vi "Read VI Ref.vi"(8 "error in (no error)":errorcluster, 11 "Graph in":refnum<class "Graph.lvclass">) -> (0 "error out":errorcluster, 2 "VI Ref":refnum<vi>, 3 "Graph out":refnum<class "Graph.lvclass">)   [LabVIEW 2021, in "Graph.lvclass"]
doc: "This vi reads Graph VI Refs."
uses:
  Graph.lvclass
  Graph.lvclass/Graph.ctl
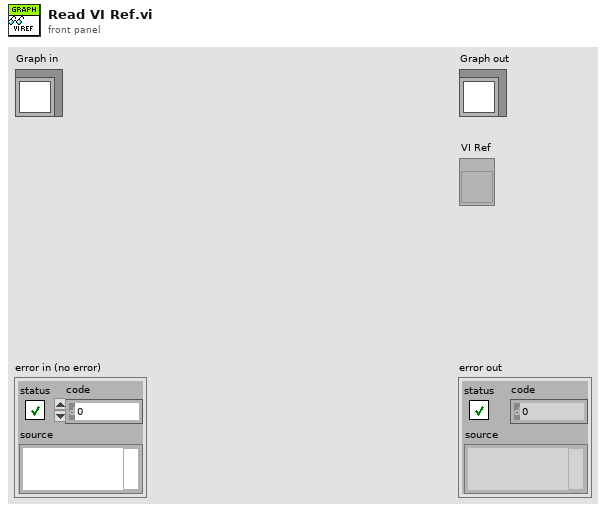
[diagram p1: front panel]
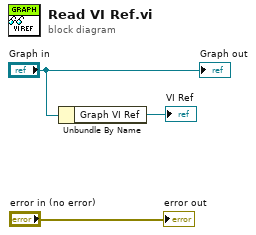
[diagram p0: block diagram]
diagram:
  n1 = Unbundle By Name("Graph in") -> ("Graph VI Ref"=→"VI Ref":refnum<vi>)
  "error out" <- "error in (no error)"
  "Graph out" <- "Graph in"
